vi "GetType.vi"(8 "error in (no error)":errorcluster, 11 "Mute All Msg":refnum<class "Mute All Msg.lvclass">) -> (0 "error out":errorcluster, 2 "Data Sample":variant, 3 "Mute All Msg":refnum<class "Mute All Msg.lvclass">)   [LabVIEW 2015, in "KIT-QVA.lvlib" / "Mute All Msg.lvclass"]
doc: "This VI delivers a sample of the data type format the message expects."
uses:
  Mute All Msg.lvclass
  Mute All Msg.lvclass/Mute All Msg.ctl
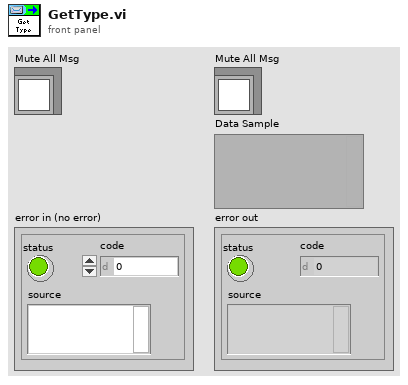
[diagram p1: front panel]
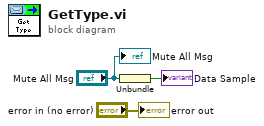
[diagram p0: block diagram]
diagram:
  n1 = Unbundle("Mute All Msg") -> (→"Data Sample":bool)
  "error out" <- "error in (no error)"
  "Mute All Msg" <- "Mute All Msg"
